vi "Read Message.vi"(8 "error in (no error)":errorcluster, 11 "abs_Log in":refnum<class "bt_Log.lvclass">) -> (0 "error out":errorcluster, 2 "Message":string, 3 "abs_Log out":refnum<class "bt_Log.lvclass">)   [LabVIEW 2021, in "BT.lvlib" / "bt_Log.lvclass"]
uses:
  bt_Log.lvclass
  bt_Log.lvclass/bt_Log.ctl
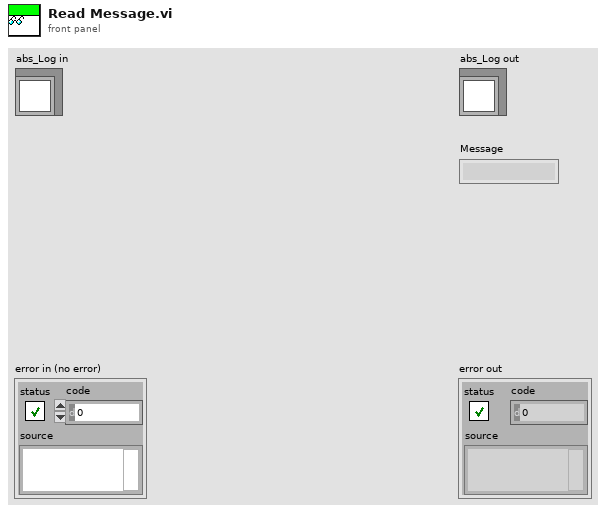
[diagram p1: front panel]
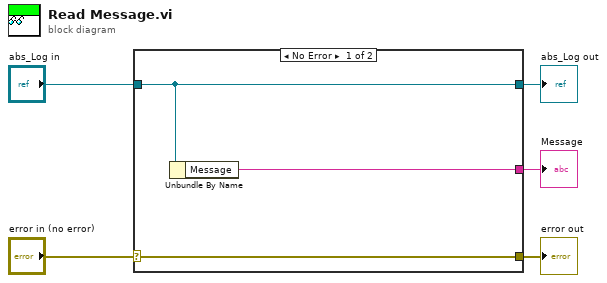
[diagram p0: block diagram]
diagram:
  n1 = case shown="No Error" "error in (no error)" {
    selector: "error in (no error)" -> [w8 w9]
    tunnel: [w8 w9] -> w4
    tunnel: [w7 w10] -> w2
    tunnel: "abs_Log in" -> [w7 w10]
    tunnel: [w6 _] -> w1
    frame No Error {
      n2 = Unbundle By Name(w7) -> ("Message"=w6:string)
    }
    frame Error {
    }
  }
  "error out" <- w4
  "abs_Log out" <- w2
  "Message" <- w1
